vi "Scan Engine Rename Slot.vi"(8 "error in (no error)":errorcluster, 9 "Name reference":refnum<vi>, 10 "Module Model":T2, 11 "Node Ptr In":T1 format="%.0x") -> (0 "error out":errorcluster, 3 "Node Ptr Out":T1 format="%.0x")   [LabVIEW 2019, in "SEECD System Explorer.lvlib"]
uses:
  SEECD System Explorer.lvlib
  Includes/Modules.lvlibp/RSI Module/Module Models.ctl
  <vilib>/NI VeriStand/Custom Device API/Custom Device Item Ref.ctl
  Includes/Modules.lvlibp/RSI Module/RSI Module.lvclass
  <vilib>/NI VeriStand/Custom Device API/Custom Device API.lvlib
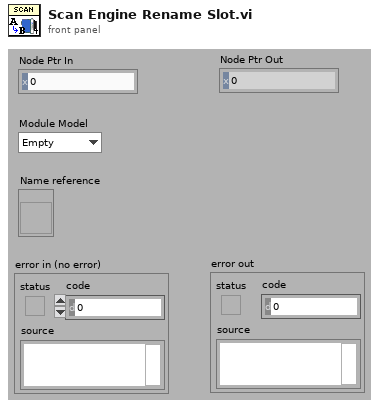
[diagram p1: front panel]
types:
  T1 = typedef "Custom Device API.lvlib/Custom Device Item Ref.ctl" = u64
  T2 = typedef "Modules.lvlibp/RSI Module.lvclass/Module Models.ctl" = enum16{"Empty", "NI 9201", "NI 9203", "NI 9205", "NI 9206", "NI 9207", "NI 9208", "NI 9209", "NI 9210", "NI 9211", "NI 9212", "NI 9213", "NI 9214", "NI 9215", "NI 9216", "NI 9217", "NI 9219", "NI 9220", "NI 9221", "NI 9222", "NI 9223", "NI 9224", "NI 9225", "NI 9226", "NI 9227", "NI 9228", "NI 9229", "NI 9233", "NI 9234", "NI 9235", "NI 9236", "NI 9237", "NI 9239", "NI 9242", "NI 9244", "NI 9253", "NI 9263", "NI 9264", "NI 9265", "NI 9266", "NI 9269", "NI 9344", "NI 9350", "NI 9375", "NI 9401", "NI 9402", "NI 9403", "NI 9411", "NI 9421", "NI 9422", "NI 9423", "NI 9425", "NI 9426", "NI 9435", "NI 9436", "NI 9437", "NI 9472", "NI 9474", "NI 9475", "NI 9476", "NI 9477", "NI 9478", "NI 9481", "NI 9482", "NI 9485"}
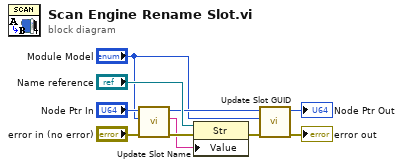
[diagram p0: block diagram]
diagram:
  n1 = call "Update Slot Name.vi"("error in"="error in (no error)", "module"="Module Model", "slot ref in"="Node Ptr In") -> ("error out"=w8:errorcluster, "name"=w4:string, "slot ref out"=w2:T1)  [unwired: 6 in]
  n2 = property class="Str"(reference="Name reference", error in=w8, "Value"=w4) -> (error out=w3:errorcluster)  [unwired: 1 out]
  n3 = call "Update Slot GUID.vi"("error in"=w3, "module model"="Module Model", "slot ref in"=w2) -> ("error out"=→"error out":errorcluster, "slot ref out"=→"Node Ptr Out":T1)  [unwired: 7 in]
